vi "ValidateDirectoryPath.vi"(8 "error in (no error)":errorcluster, 11 "MassCompile in":refnum<class "MassCompile.lvclass">) -> (0 "error out":errorcluster, 3 "MassCompile out":refnum<class "MassCompile.lvclass">)   [LabVIEW 2014, in "MassCompile.lvclass"]
uses:
  MassCompile.lvclass
  MassCompile.lvclass/MassCompile.ctl
  Utilities/OperationErrorType.ctl
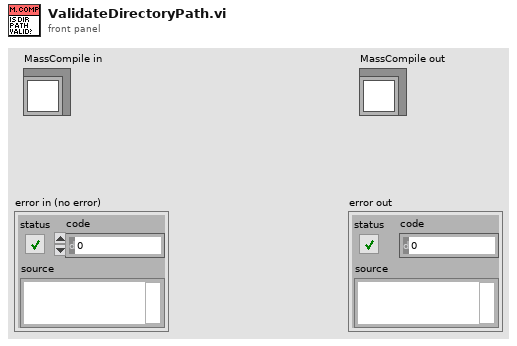
[diagram p1: front panel]
types:
  T1 = typedef "OperationErrorType.ctl" = enum16{"RequiredArgumentMissing", "UnknownArguments", "LoggerSetMultipleTimes", "OperationBrokenError"}
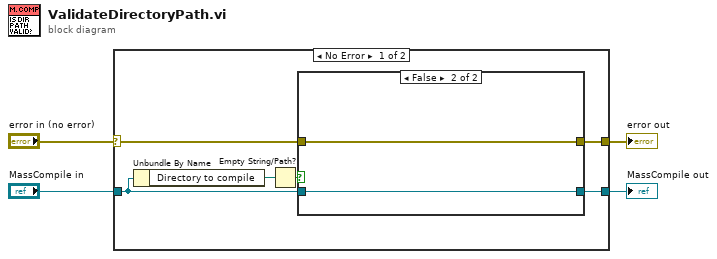
[diagram p0: block diagram]
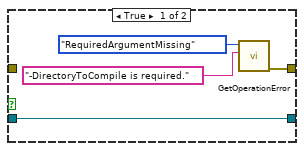
[diagram p2: hidden frame]
diagram:
  n1 = case shown="No Error" "error in (no error)" {
    selector: "error in (no error)" -> [w5 w18]
    tunnel: [w10 w18] -> w4
    tunnel: "MassCompile in" -> [w7 w17]
    tunnel: [w6 w17] -> w2
    frame No Error {
      n2 = Unbundle By Name(w7) -> ("Directory to compile"=w8:path)
      n3 = Empty String/Path?(string/path=w8) -> (empty?=w9:bool)
      n4 = case shown="False" w9 {
        tunnel: w5 -> [_ w16]
        tunnel: [w13 w16] -> w10
        tunnel: w7 -> [w14 w15]
        tunnel: [w14 w15] -> w6
        frame True {
          n5 = call "GetOperationError.vi"("Additional Information"="-DirectoryToCompile is required.", "Operation Error Type"=OperationErrorType."RequiredArgumentMissing") -> ("error out"=w13:errorcluster)  [unwired: 9 in]
        }
        frame False {
        }
      }
    }
    frame Error {
    }
  }
  "error out" <- w4
  "MassCompile out" <- w2
